vi "Inline Read All.vi"(8 "error in (no error)":errorcluster, 11 "uData in":refnum<class "uData.lvclass">) -> (0 "error out":errorcluster, 1 "values":variant[](array[variant]), 2 "keys":string[](array[string]), 3 "uData out":refnum<class "uData.lvclass">)   [LabVIEW 2023, in "uLib.lvlib" / "uData.lvclass"]
doc: "Dynamic dispatch method to list all available tags/keys and their values.\n\n<B>THE \"INLINE\" DYNAMIC DISPATCH METHOD GROUP ARE THE ONLY METHODS THAT ARE ALLOWED TO ACCESS THE OBJECT PRIVATE DATA.</B>\n\nCONVERTED TO INLINE STATIC DISPATCH TO MITIGATE THE PERFORMANCE OVERHEAT HIT REALIZED IN INTIAL TESTING."
uses:
  uData.lvclass
  uData.lvclass/uData.ctl
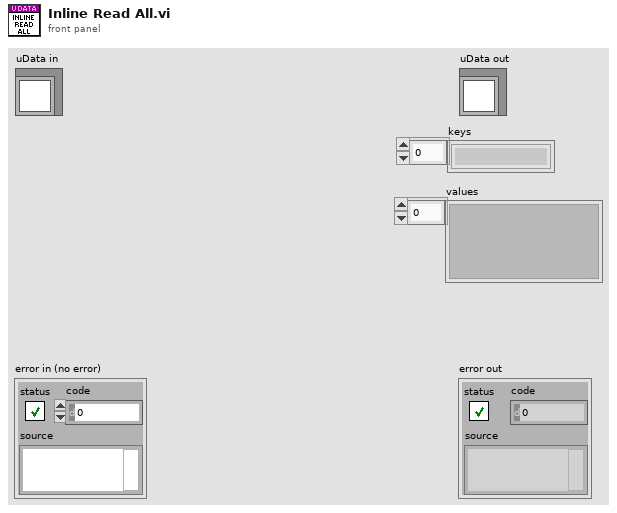
[diagram p1: front panel]
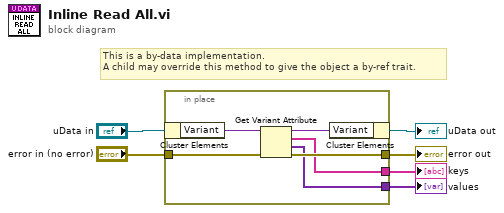
[diagram p0: block diagram]
diagram:
  # "This is a by-data implementation.\nA child may override this method to give the object a by-ref trait."
  n1 = in-place {
    in-place-border: [w10] -> w5
    in-place-border: "error in (no error)" -> [w9]
    in-place-border: [w8] -> w2
    in-place-border: [w7] -> w1
    n2 = in-place-cluster #1("uData in") -> ("Variant"=w12:variant)
    n3 = Get Variant Attribute(Variant=w12, error in=w9) -> (duplicate Variant=w11:variant, names=w8:string[], values=w7:variant[], error out=w10:errorcluster)  [unwired: 2 in]
    n4 = in-place-cluster #1("Variant"=w11) -> (→"uData out":refnum<class "uData.lvclass">)
  }
  "error out" <- w5
  "keys" <- w2
  "values" <- w1
